vi "DoNanoOpSendCmdNoResp.vi"(8 "error in (no error)":errorcluster, 9 "1sec delay after?":bool=TRUE, 10 "Cmd String":string, 11 "VISA resource name":refnum<visa-resource-name>) -> (0 "error out":errorcluster, 3 "VISA resource name out":refnum<visa-resource-name>)   [LabVIEW 2013]
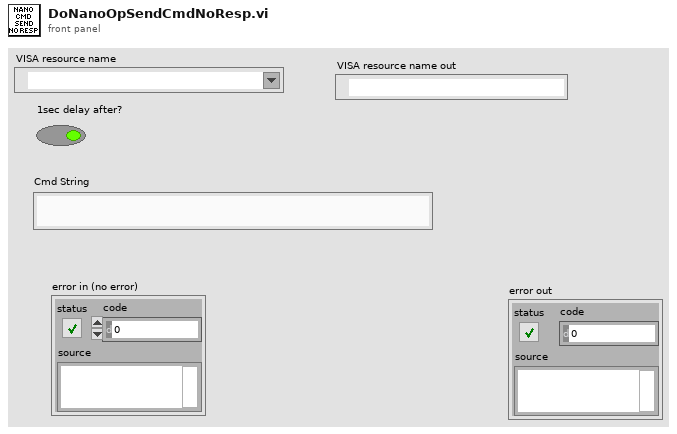
[diagram p1: front panel]
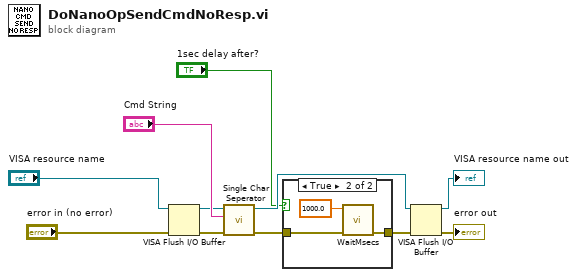
[diagram p0: block diagram]
diagram:
  n1 = VISA Flush I/O Buffer(VISA resource name="VISA resource name", error in (no error)="error in (no error)") -> (VISA resource name out=w5:refnum<visa-resource-name>, error out=w6:errorcluster)  [unwired: 1 in]
  n2 = call "Single Char Seperator.vi"("error in (no error)"=w6, "String"="Cmd String", "VISA resource name"=w5) -> ("error out"=w3:errorcluster, "VISA resource name 2"=w4:refnum<visa-resource-name>)  [unwired: 7 in]
  n3 = case shown="True" "1sec delay after?" {
    tunnel: w3 -> [w12 w15]
    tunnel: [w12 w14] -> w2
    frame False {
    }
    frame True {
      n4 = call "WaitMsecs.vi"("error in (no error)"=w15, "Wait Msecs"=1000.0) -> ("error out"=w14:errorcluster)  [unwired: 9 in]
    }
  }
  n5 = VISA Flush I/O Buffer(VISA resource name=w4, error in (no error)=w2) -> (VISA resource name out=→"VISA resource name out":refnum<visa-resource-name>, error out=→"error out":errorcluster)  [unwired: 1 in]
